vi "Control Drive with Limelight.vi"(9 "X-DriveAuto":dbl, 11 "Y-DriveAuto":dbl) -> ()   [LabVIEW 2020]
uses:
  Framework/Robot Global Data.vi
  <vilib>/Rock Robotics/WPI/Utilities/WPI_GetSetVariantRefNum.vi
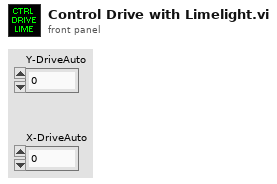
[diagram p1: front panel]
types:
  T1 = typedef "WPI_RobotDriveDevRef.ctl" = cluster{"DevStatus":errorcluster, "Motors[]":T2[], "Square Inputs":bool, "Max Output":dbl}
  T2 = typedef "WPI_MotorControlDeviceRef.ctl" = cluster{"DeviceStatus":errorcluster, "Type":T3, "PWM":cluster{"PWM Channel":T4, "DeadBand":T5}, "CAN":cluster{"Device Number":u8, "SetOutput VI Ref":variant, "GetOutput VI Ref":variant, "Enable VI Ref":variant, "Disable VI Ref":variant, "Data":variant}, "Invert":bool, "DIO PWM":cluster{"PWM \"Enable\" Channel":T4, "DIOChannel":T6, "PWM Rate":dbl}}
  T3 = typedef "WPI_MotorControlType.ctl" = enum16{"PWM", "CAN", "DIO PWM"}
  T4 = typedef "FPGA_DIOPWMChannel.ctl" = enum8{"PWM 0", "PWM 1", "PWM 2", "PWM 3", "PWM 4", "PWM 5", "PWM 6", "PWM 7", "PWM 8", "PWM 9", "PWM MXP 0", "PWM MXP 1", "PWM MXP 2", "PWM MXP 3", "PWM MXP 4", "PWM MXP 5", "PWM MXP 6", "PWM MXP 7", "PWM MXP 8", "PWM MXP 9", "Invalid"}
  T5 = typedef "WPI_PWMDeadband.ctl" = cluster{"Name":string, "maxPositivePwm":i32, "minPositivePwm":i32, "centerPwm":i32, "maxNegativePwm":i32, "minNegativePwm":i32, "angularRange":u16}
  T6 = typedef "FPGA_DIOChannel.ctl" = enum8{"DIO 0", "DIO 1", "DIO 2", "DIO 3", "DIO 4", "DIO 5", "DIO 6", "DIO 7", "DIO 8", "DIO 9", "DIO MXP 0", "DIO MXP 1", "DIO MXP 2", "DIO MXP 3", "DIO MXP 4", "DIO MXP 5", "DIO MXP 6", "DIO MXP 7", "DIO MXP 8", "DIO MXP 9", "DIO MXP 10", "DIO MXP 11", "DIO MXP 12", "DIO MXP 13", "DIO MXP 14", "DIO MXP 15", "SPI Port CS1", "SPI Port CS2", "SPI Port CS3", "SPI Port MISO", "SPI Port MOSI", "Invalid"}
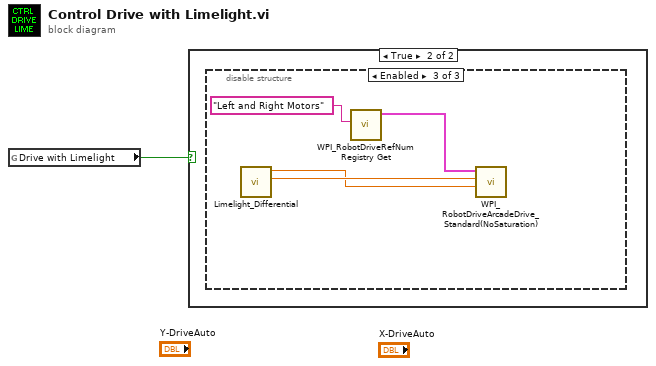
[diagram p0: block diagram]
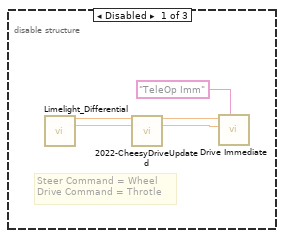
[diagram p3: hidden frame]
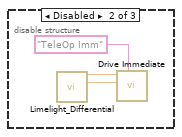
[diagram p4: hidden frame]
diagram:
  n1 = global read "Robot Global Data.vi" "Drive with Limelight"() -> (w1:bool)
  n2 = case shown="True" w1 {
    frame False {
    }
    frame True {
      n3 = disable-structure shown="Enabled" {
        frame Disabled {
          # "Steer Command = Wheel\nDrive Command = Throtle"
          n4 = call "Limelight_Differential.vi"() -> ("SteerCommand"=w2:dbl, "DriveCommand"=w3:dbl)  [unwired: 8 in, 1 out]
          n5 = call "2022-CheesyDriveUpdated.vi"("Throttle"=w3, "Wheel"=w2) -> ("Left PWM"=w5:dbl, "Right PWM"=w4:dbl)  [unwired: 12 in]
          n6 = call "Drive Immediate.vi"("Description"="TeleOp Imm", "Right Setpoint"=w4, "Left Setpoint"=w5) -> ()  [unwired: 8 in, 1 out]
        }
        frame Disabled {
          n7 = call "Limelight_Differential.vi"() -> ("SteerCommand"=w7:dbl, "DriveCommand"=w8:dbl)  [unwired: 8 in, 1 out]
          n8 = call "Drive Immediate.vi"("Description"="TeleOp Imm", "Right Setpoint"=w7, "Left Setpoint"=w8) -> ()  [unwired: 8 in, 1 out]
        }
        frame Enabled {
          n9 = call "Limelight_Differential.vi"() -> ("SteerCommand"=w11:dbl, "DriveCommand"=w10:dbl)  [unwired: 8 in, 1 out]
          n10 = call <vilib>:"WPI_RobotDriveRefNum Registry Get.vi"("refnum name"="Left and Right Motors") -> ("RobotDriveDevRef"=w12:T1)  [unwired: 9 in, 1 out]
          n11 = call <vilib>:"WPI_RobotDriveArcadeDrive_Standard(NoSaturation).vi"("Y axis value"=w10, "X axis value"=w11, "RobotDriveDevRef"=w12) -> ()  [unwired: 1 in, 8 out]
        }
      }
    }
  }
